vi "OPC Tags.vi"(11 "OPC Module Configs":T1[](array[typedef]) {"Data"."Variable Array"."status" items=["Good"=0, "Good_SubscriptionTransferred"=2949120, "Good_CompletesAsynchronously"=3014656, "Good_Overload"=3080192, "Good_Clamped"=3145728, "Good_LocalOverride"=9830400, "Good_EntryInserted"=10616832, "Good_EntryReplaced"=10682368, "Good_NoData"=10813440, "Good_MoreData"=10878976, "Good_CommunicationEvent"=10944512, "Good_ShutdownEvent"=11010048, "Good_CallAgain"=11075584, "Good_NonCriticalTimeout"=11141120, "Good_ResultsMayBeIncomplete"=12189696, "Good_DataIgnored"=14221312, "Uncertain"=1073741824, "Uncertain_ReferenceOutOfServer"=1080819712, "Uncertain_NoCommunicationLastUsableValue"=1083113472, "Uncertain_LastUsableValue"=1083179008, "Uncertain_SubstituteValue"=1083244544, "Uncertain_InitialValue"=1083310080, "Uncertain_SensorNotAccurate"=1083375616, "Uncertain_EngineeringUnitsExceeded"=1083441152, "Uncertain_SubNormal"=1083506688, "Uncertain_DataSubNormal"=1084489728, "Uncertain_ReferenceNotDeleted"=1086062592, "Uncertain_NotAllNodesAvailable"=1086324736, "Bad"=2147483648, "Bad_UnexpectedError"=2147549184, "Bad_InternalError"=2147614720, "Bad_OutOfMemory"=2147680256, "Bad_ResourceUnavailable"=2147745792, "Bad_CommunicationError"=2147811328, "Bad_EncodingError"=2147876864, "Bad_DecodingError"=2147942400, "Bad_EncodingLimitsExceeded"=2148007936, "Bad_UnknownResponse"=2148073472, "Bad_Timeout"=2148139008, "Bad_ServiceUnsupported"=2148204544, "Bad_Shutdown"=2148270080, "Bad_ServerNotConnected"=2148335616, "Bad_ServerHalted"=2148401152, "Bad_NothingToDo"=2148466688, "Bad_TooManyOperations"=2148532224, "Bad_DataTypeIdUnknown"=2148597760, "Bad_CertificateInvalid"=2148663296, "Bad_SecurityChecksFailed"=2148728832, "Bad_CertificateTimeInvalid"=2148794368, "Bad_CertificateIssuerTimeInvalid"=2148859904, "Bad_CertificateHostNameInvalid"=2148925440, "Bad_CertificateUriInvalid"=2148990976, "Bad_CertificateUseNotAllowed"=2149056512, "Bad_CertificateIssuerUseNotAllowed"=2149122048, "Bad_CertificateUntrusted"=2149187584, "Bad_CertificateRevocationUnknown"=2149253120, "Bad_CertificateIssuerRevocationUnknown"=2149318656, "Bad_CertificateRevoked"=2149384192, "Bad_CertificateIssuerRevoked"=2149449728, "Bad_UserAccessDenied"=2149515264, "Bad_IdentityTokenInvalid"=2149580800, "Bad_IdentityTokenRejected"=2149646336, "Bad_SecureChannelIdInvalid"=2149711872, "Bad_InvalidTimestamp"=2149777408, "Bad_NonceInvalid"=2149842944, "Bad_SessionIdInvalid"=2149908480, "Bad_SessionClosed"=2149974016, "Bad_SessionNotActivated"=2150039552, "Bad_SubscriptionIdInvalid"=2150105088, "Bad_RequestHeaderInvalid"=2150236160, "Bad_TimestampsToReturnInvalid"=2150301696, "Bad_RequestCancelledByClient"=2150367232, "Bad_NoCommunication"=2150694912, "Bad_WaitingForInitialData"=2150760448, "Bad_NodeIdInvalid"=2150825984, "Bad_NodeIdUnknown"=2150891520, "Bad_AttributeIdInvalid"=2150957056, "Bad_IndexRangeInvalid"=2151022592, "Bad_IndexRangeNoData"=2151088128, "Bad_DataEncodingInvalid"=2151153664, "Bad_DataEncodingUnsupported"=2151219200, "Bad_NotReadable"=2151284736, "Bad_NotWritable"=2151350272, "Bad_OutOfRange"=2151415808, "Bad_NotSupported"=2151481344, "Bad_NotFound"=2151546880, "Bad_ObjectDeleted"=2151612416, "Bad_NotImplemented"=2151677952, "Bad_MonitoringModeInvalid"=2151743488, "Bad_MonitoredItemIdInvalid"=2151809024, "Bad_MonitoredItemFilterInvalid"=2151874560, "Bad_MonitoredItemFilterUnsupported"=2151940096, "Bad_FilterNotAllowed"=2152005632, "Bad_StructureMissing"=2152071168, "Bad_EventFilterInvalid"=2152136704, "Bad_ContentFilterInvalid"=2152202240, "Bad_FilterOperandInvalid"=2152267776, "Bad_ContinuationPointInvalid"=2152333312, "Bad_NoContinuationPoints"=2152398848, "Bad_ReferenceTypeIdInvalid"=2152464384, "Bad_BrowseDirectionInvalid"=2152529920, "Bad_NodeNotInView"=2152595456, "Bad_ServerUriInvalid"=2152660992, "Bad_ServerNameMissing"=2152726528, "Bad_DiscoveryUrlMissing"=2152792064, "Bad_SempahoreFileMissing"=2152857600, "Bad_RequestTypeInvalid"=2152923136, "Bad_SecurityModeRejected"=2152988672, "Bad_SecurityPolicyRejected"=2153054208, "Bad_TooManySessions"=2153119744, "Bad_UserSignatureInvalid"=2153185280, "Bad_ApplicationSignatureInvalid"=2153250816, "Bad_NoValidCertificates"=2153316352, "Bad_RequestCancelledByRequest"=2153381888, "Bad_ParentNodeIdInvalid"=2153447424, "Bad_ReferenceNotAllowed"=2153512960, "Bad_NodeIdRejected"=2153578496, "Bad_NodeIdExists"=2153644032, "Bad_NodeClassInvalid"=2153709568, "Bad_BrowseNameInvalid"=2153775104, "Bad_BrowseNameDuplicated"=2153840640, "Bad_NodeAttributesInvalid"=2153906176, "Bad_TypeDefinitionInvalid"=2153971712, "Bad_SourceNodeIdInvalid"=2154037248, "Bad_TargetNodeIdInvalid"=2154102784, "Bad_DuplicateReferenceNotAllowed"=2154168320, "Bad_InvalidSelfReference"=2154233856, "Bad_ReferenceLocalOnly"=2154299392, "Bad_NoDeleteRights"=2154364928, "Bad_ServerIndexInvalid"=2154430464, "Bad_ViewIdUnknown"=2154496000, "Bad_TooManyMatches"=2154627072, "Bad_QueryTooComplex"=2154692608, "Bad_NoMatch"=2154758144, "Bad_MaxAgeInvalid"=2154823680, "Bad_HistoryOperationInvalid"=2154889216, "Bad_HistoryOperationUnsupported"=2154954752, "Bad_WriteNotSupported"=2155020288, "Bad_TypeMismatch"=2155085824, "Bad_MethodInvalid"=2155151360, "Bad_ArgumentsMissing"=2155216896, "Bad_TooManySubscriptions"=2155282432, "Bad_TooManyPublishRequests"=2155347968, "Bad_NoSubscription"=2155413504, "Bad_SequenceNumberUnknown"=2155479040, "Bad_MessageNotAvailable"=2155544576, "Bad_InsufficientClientProfile"=2155610112, "Bad_TcpServerTooBusy"=2155675648, "Bad_TcpMessageTypeInvalid"=2155741184, "Bad_TcpSecureChannelUnknown"=2155806720, "Bad_TcpMessageTooLarge"=2155872256, "Bad_TcpNotEnoughResources"=2155937792, "Bad_TcpInternalError"=2156003328, "Bad_TcpEndpointUrlInvalid"=2156068864, "Bad_RequestInterrupted"=2156134400, "Bad_RequestTimeout"=2156199936, "Bad_SecureChannelClosed"=2156265472, "Bad_SecureChannelTokenUnknown"=2156331008, "Bad_SequenceNumberInvalid"=2156396544, "Bad_ConfigurationError"=2156462080, "Bad_NotConnected"=2156527616, "Bad_DeviceFailure"=2156593152, "Bad_SensorFailure"=2156658688, "Bad_OutOfService"=2156724224, "Bad_DeadbandFilterInvalid"=2156789760, "Bad_RefreshInProgress"=2157379584, "Bad_ConditionAlreadyDisabled"=2157445120, "Bad_ConditionDisabled"=2157510656, "Bad_EventIdUnknown"=2157576192, "Bad_NoData"=2157641728, "Bad_DataLost"=2157772800, "Bad_DataUnavailable"=2157838336, "Bad_EntryExists"=2157903872, "Bad_NoEntryExists"=2157969408, "Bad_TimestampNotSupported"=2158034944, "Bad_InvalidArgument"=2158690304, "Bad_ConnectionRejected"=2158755840, "Bad_Disconnect"=2158821376, "Bad_ConnectionClosed"=2158886912, "Bad_InvalidState"=2158952448, "Bad_EndOfStream"=2159017984, "Bad_NoDataAvailable"=2159083520, "Bad_WaitingForResponse"=2159149056, "Bad_OperationAbandoned"=2159214592, "Bad_ExpectedStreamToBlock"=2159280128, "Bad_WouldBlock"=2159345664, "Bad_SyntaxError"=2159411200, "Bad_MaxConnectionsReached"=2159476736, "Bad_RequestTooLarge"=2159542272, "Bad_ResponseTooLarge"=2159607808, "Bad_EventNotAcknowledgeable"=2159738880, "Bad_InvalidTimestampArgument"=2159869952, "Bad_ProtocolVersionUnsupported"=2159935488, "Bad_StateNotActive"=2160001024, "Bad_FilterOperatorInvalid"=2160132096, "Bad_FilterOperatorUnsupported"=2160197632, "Bad_FilterOperandCountMismatch"=2160263168, "Bad_FilterElementInvalid"=2160328704, "Bad_FilterLiteralInvalid"=2160394240, "Bad_IdentityChangeNotSupported"=2160459776, "Bad_NotTypeDefinition"=2160590848, "Bad_ViewTimestampInvalid"=2160656384, "Bad_ViewParameterMismatch"=2160721920, "Bad_ViewVersionInvalid"=2160787456, "Bad_ConditionAlreadyEnabled"=2160852992, "Bad_DialogNotActive"=2160918528, "Bad_DialogResponseInvalid"=2160984064, "Bad_ConditionBranchAlreadyAcked"=2161049600, "Bad_ConditionBranchAlreadyConfirmed"=2161115136, "Bad_ConditionAlreadyShelved"=2161180672, "Bad_ConditionNotShelved"=2161246208, "Bad_ShelvingTimeOutOfRange"=2161311744, "Bad_AggregateListMismatch"=2161377280, "Bad_AggregateNotSupported"=2161442816, "Bad_AggregateInvalidInputs"=2161508352, "Bad_BoundNotFound"=2161573888, "Bad_BoundNotSupported"=2161639424, "Bad_AggregateConfigurationRejected"=2161770496, "Bad_TooManyMonitoredItems"=2161836032]}) -> (1 "OPC Tags":T11, 2 "OPC Module Tags Array":T10(array[cluster]), 3 "All Boolean Tags 7":string[](array[string]), 4 "All  Numeric Tags 7":string[](array[string]))   [LabVIEW 2018]
uses:
  OPC Module Config.ctl
  Scale Module Folder/Measure Instrument/State Enum.ctl
  <vilib>/Utility/miscctls.llb/LVPoint32TypeDef.ctl
  OPC Settings.ctl
  Variable Data Cluster.ctl
  <vilib>/OPCUA/controls/NodeId.ctl
  <vilib>/OPCUA/controls/OPC UA StatusCode.ctl
  <vilib>/OPCUA/controls/Subscription ID.ctl
  <vilib>/OPCUA/controls/OPC UA Client Refnum.ctl
  <vilib>/OPCUA/controls/Subscription Data Change.ctl
  <vilib>/OPCUA/controls/Data Type.ctl
  OPC UA.lvlib
  Scale Module Folder/Measure Instrument/Scale Module Engine.lvlib
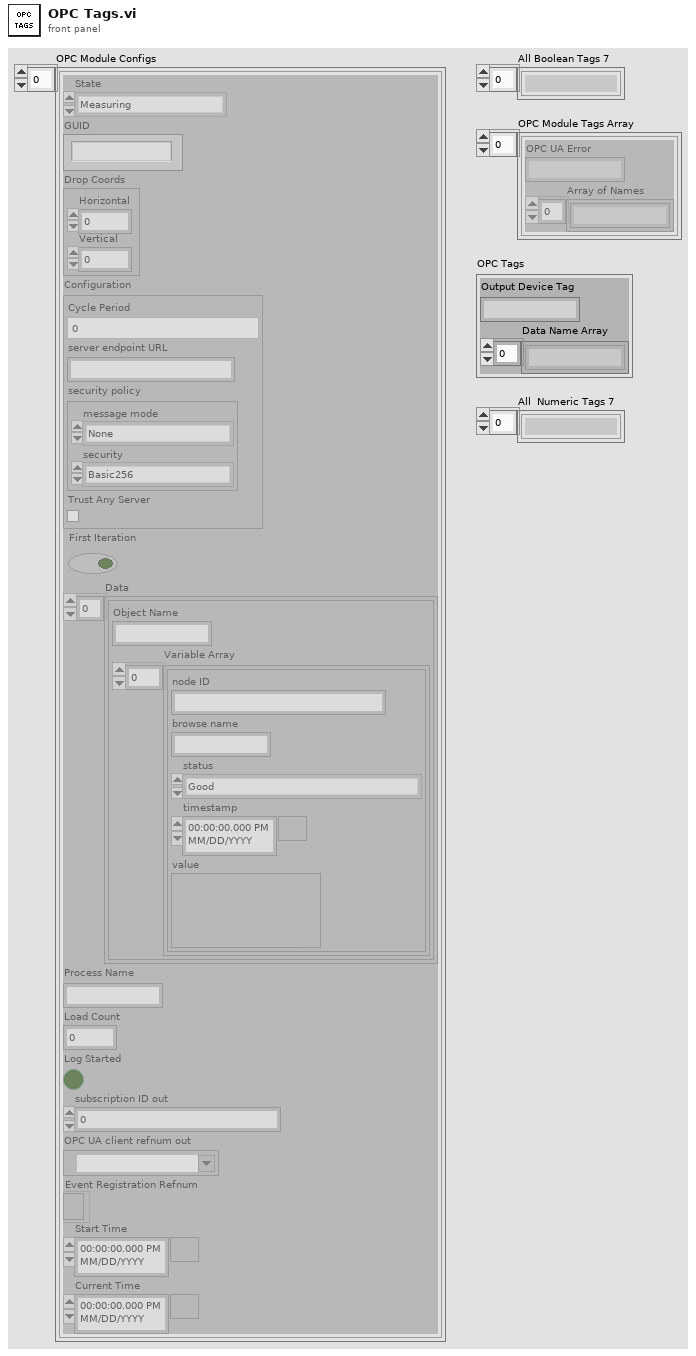
[diagram p1: front panel]
types:
  T1 = typedef "OPC UA.lvlib/OPC Module Config.ctl" = cluster{"State":T2, "GUID":string, "Drop Coords":T3, "Configuration":T4, "First Iteration":bool, "Data":cluster{"Object Name":string, "Variable Array":T5[]}[], "Process Name":string, "Load Count":i32, "Log Started":bool, "subscription ID out":T8, "OPC UA client refnum out":T9, "Event Registration Refnum":refnum<event-registration>, "Start Time":timestamp, "Current Time":timestamp}
  T2 = typedef "Scale Module.lvlib/Scale Module Engine.lvlib/State Enum.ctl" = enum16{"Measuring", "Idle"}
  T3 = typedef "LVPoint32TypeDef.ctl" = cluster{"Horizontal":i32, "Vertical":i32}
  T4 = typedef "OPC UA.lvlib/OPC Settings.ctl" = cluster{"Cycle Period":dbl, "server endpoint URL":string, "security policy":cluster{"message mode":enum16{"None", "Sign", "Sign and Encrypt"}, "security":enum16{"Basic256", "Basic128Rsa15"}}, "Trust Any Server":bool}
  T5 = typedef "OPC UA.lvlib/Variable Data Cluster.ctl" = cluster{"node ID":T6, "browse name":string, "status":T7, "timestamp":timestamp, "value ":variant}
  T6 = typedef "NodeId.ctl" = string
  T7 = typedef "OPC UA StatusCode.ctl" = u32
  T8 = typedef "Subscription ID.ctl" = u32
  T9 = typedef "OPC UA Client Refnum.ctl" = refnum<k21>
  T10 = cluster{"OPC UA Error":string, "Array of Names":string[]}[]
  T11 = cluster{"Output Device Tag":string, "Data Name Array":string[]}
  T12 = cluster{"OPC UA Error":string, "Array of Names":string[]}
  T13 = cluster{"Object Name":string, "Variable Array":T5[]}[]
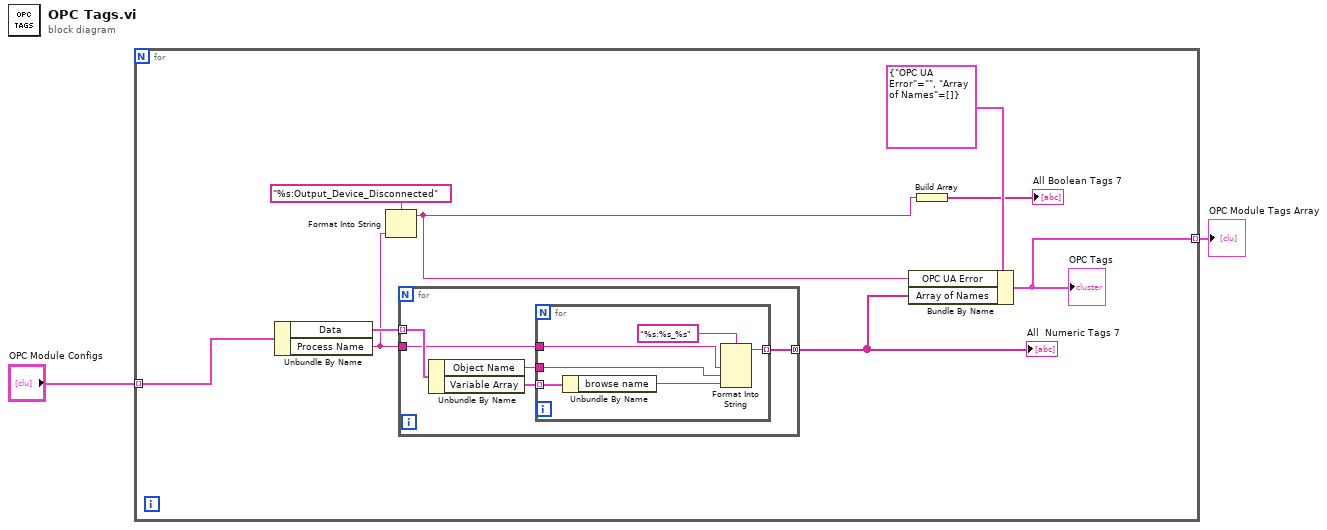
[diagram p0: block diagram]
diagram:
  n1 = for {
    tunnel: "OPC Module Configs" -> [w4] mode=indexing
    tunnel: [w3] -> w2 mode=indexing
    n2 = Unbundle By Name(w4) -> ("Data"=w7:T13, "Process Name"=w6:string)
    n3 = Format Into String(format string="%s:Output_Device_Disconnected", w6) -> (resulting string=w9:string)  [unwired: 2 in, 1 out]
    n4 = for {
      tunnel: w7 -> [w16] mode=indexing
      tunnel: w6 -> [w13]
      tunnel: [w12] -> w5 mode=concatenating
      n5 = Unbundle By Name(w16) -> ("Object Name"=w14:string, "Variable Array"=w15:T5[])
      n6 = for {
        tunnel: w15 -> [w18] mode=indexing
        tunnel: w14 -> [w19]
        tunnel: w13 -> [w21]
        tunnel: [w20] -> w12 mode=indexing
        n7 = Unbundle By Name(w18) -> ("browse name"=w17:string)
        n8 = Format Into String(format string="%s:%s_%s", w21, w19, w17) -> (resulting string=w20:string)  [unwired: 2 in, 1 out]
      }
    }
    "All  Numeric Tags 7" <- w5
    n9 = Bundle By Name(cluster=T12 {"OPC UA Error"="", "Array of Names"=[]} ("Scale Tags 2"), "OPC UA Error"=w9, "Array of Names"=w5) -> (w3:T12)
    "OPC Tags" <- w3
    n10 = Build Array(w9) -> (→"All Boolean Tags 7":string[])
  }
  "OPC Module Tags Array" <- w2
